vi "Minimise.vi"(8 "error in (no error)":errorcluster, 11 "module in":refnum<class "TitleBar.lvclass">) -> (0 "error out":errorcluster, 3 "module out":refnum<class "TitleBar.lvclass">)   [LabVIEW 2024, in "TitleBar.lvclass"]
uses:
  TitleBar.lvclass
  Minimise.ctl
  RQMHCore/ModuleCore/RQMHModule.lvclass
  TitleBar.lvclass/TitleBar.ctl
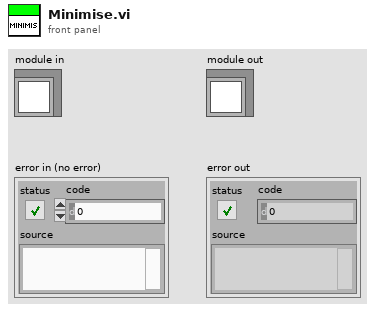
[diagram p1: front panel]
types:
  T1 = typedef "TitleBar.lvclass/Minimise.ctl" = cluster{"Module":refnum<class "RQMHModule.lvclass">, "null":bool}
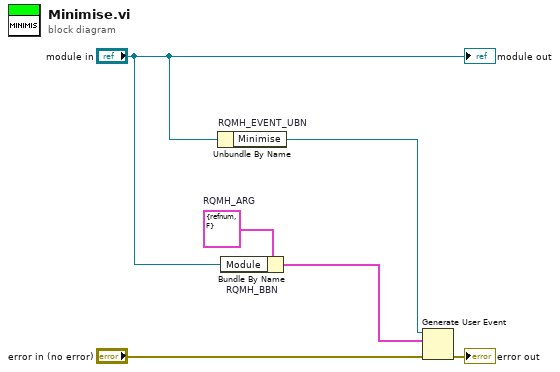
[diagram p0: block diagram]
diagram:
  w3 = T1 {"Module"=refnum, "null"=FALSE}  # RQMH_ARG
  n1 = Unbundle By Name "RQMH_EVENT_UBN"("module in") -> ("Minimise"=w6:refnum<user-event>)
  n2 = Bundle By Name "RQMH_BBN"(cluster=w3, "Module"="module in") -> (w2:T1)
  n3 = Generate User Event(user event=w6, event data cluster=w2, error in="error in (no error)") -> (error out=→"error out":errorcluster)  [unwired: 1 in, 1 out]
  "module out" <- "module in"
